vi "Exp11.vi"() -> ()   [LabVIEW 2009]
uses:
  <vilib>/Simulation/Scripting/Companion Diagram/SimConfigNode/SimDog.xnode
  <vilib>/Simulation/Scripting/Companion Diagram/SimConfigNode/SimParams.ctl
  <vilib>/Simulation/Scripting/Companion Diagram/SimConfigNode/_simSolvers.ctl
  <vilib>/Simulation/Implementation/Shared/SIMSCR Execution Mode.ctl
  <vilib>/Simulation/Implementation/Shared/SIM Bundle Sim Info.vi
  <vilib>/Simulation/Implementation/Shared/NILVSim_GetModelError.vi
  <vilib>/Simulation/Implementation/Shared/SIM Unbundle Sim Info.vi
  <vilib>/Platform/TimedLoop/XDataNode/XDataNode.xnode
  <vilib>/Platform/TimedLoop/XDataNode/loadlvalarms.vi
  <vilib>/Platform/TimedLoop/XDataNode/timing_clust.ctl
  <vilib>/Platform/TimedLoop/XDataNode/nitl_modes.ctl
  <vilib>/Platform/TimedLoop/XDataNode/wakeup.ctl
  <vilib>/Simulation/Implementation/Shared/NILVSim_Initialize.vi
  <vilib>/Simulation/Implementation/Shared/NILVSim_FinishedLate.vi
  <vilib>/Simulation/Implementation/Shared/NILVSim_Manager.vi
  <vilib>/Simulation/Scripting/Editor Utilities/SIM subVI tag data.ctl
  <vilib>/Simulation/Scripting/Editor Utilities/SIM subVI execution type.ctl
  <vilib>/Simulation/Utility/SIMX Halt/SIMX Halt.xnode
  <vilib>/Simulation/Utility/Implementation/SIM Halt.vi
  <vilib>/Simulation/Implementation/Shared/SIM Fire Discrete SubVI.vi
  <vilib>/Simulation/SignalArithmetic/SIMX Gain/SIMX Gain.xnode
  <vilib>/Simulation/SignalArithmetic/Implementation/NILVSim Gain.llb/SIM Gain (scalar).vi
  <vilib>/Simulation/SignalArithmetic/SIMX Summation/SIMX Summation.xnode
  <vilib>/Simulation/Nonlinear/SIMX Saturation/SIMX Saturation.xnode
  <vilib>/Simulation/Nonlinear/Implementation/NILVSim Saturation.llb/SIM Saturation (scalar).vi
  <vilib>/Simulation/Implementation/Shared/NILVSim_FinalizeModel.vi
  Instance           8 13Saved   Exp10 .vi
  Instance           9 13Saved   Exp10 .vi
  Instance          10 13Saved   Exp10 .vi
  Instance          11 13Saved   Exp10 .vi
  <vilib>/Platform/TimedLoop/XDataNode/XDNodeRunTimeDep.lvlib
panel:
  in  "Controlador":cluster{"Kc":dbl, "Kaux":dbl}
  in  "stop":bool
  in  "Set-Point":T1={"Magnitude"=5.0, "Frequência"=0.02, "Offset"=2.5}
  in  "Set-point:\nMan / Auto":bool
  out "Medidas":dbl[][](graph)
  in  "AO0\n(manual)":dbl(slide) scale=-10.0..10.0
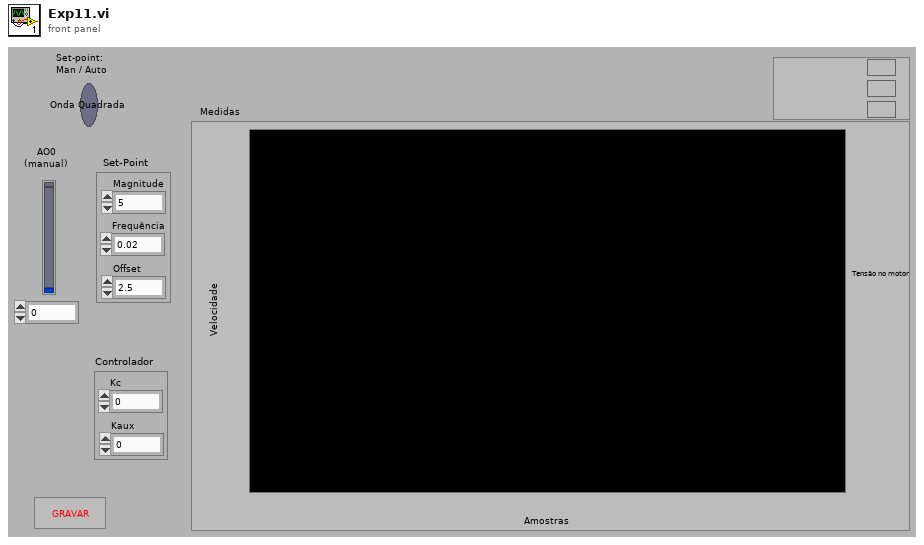
[diagram p1: front panel]
types:
  T1 = cluster{"Magnitude":dbl, "Frequência":dbl, "Offset":dbl}
  T2 = typedef "SIM subVI tag data.ctl" = cluster{"period":dbl, "skew":dbl, "Simulation execution type":T3}
  T3 = typedef "SIM subVI execution type.ctl" = enum16{"Function call", "Discrete", "Continuous", "Initialization only", "Final step only"}
  T4 = typedef "XDNodeRunTimeDep.lvlib/timing_clust.ctl" = cluster{"Expected End [f-1]":u64, "Actual End [f-1]":u64, "Finished Late? [f-1]":bool, "Expected End [i-1]":u64, "Actual End [i-1]":u64, "Finished Late? [i-1]":bool, "Expected Start [i]":u64, "Actual Start [i]":u64, "Expected Start [f]":u64, "Actual Start [f]":u64, "Source Name":string, "Structure Name":string, "Period":i64, "Deadline":i64, "Offset":i64, "Start":i64, "Priority":i32, "Timeout":i32, "Mode":T5, "Wakeup Reason":T6, "Error":errorcluster, "Source Type":string, "Secondary Source Type":string, "Global End Time":u64, "Global Start Time":u64, "Frame Duration":u64, "Iteration Duration":u64, "Assigned CPU":i32, "I/O Scan Engine Mode":u32}
  T5 = typedef "XDNodeRunTimeDep.lvlib/nitl_modes.ctl" = enum32{"No Change", "Process missed periods, maintain original phase", "Discard missed periods, maintain original phase", "Process missed periods, ignore original phase", "Discard missed periods, ignore original phase"}
  T6 = typedef "XDNodeRunTimeDep.lvlib/wakeup.ctl" = enum32{"Normal", "Aborted", "Asynchronous wakeup", "Timing source error", "Timed loop error", "Timeout"}
  T7 = typedef "SimParams.ctl" = cluster{"Initial Time (s)":dbl, "Final Time (s)":dbl, "Step Size (s)":dbl, "ODE Solver":T8, "Minimum Step Size (s)":dbl, "Maximum Step Size (s)":dbl, "Relative Tolerance":dbl, "Absolute Tolerance":dbl, "Software Timing":bool, "Initial Step Size (s)":dbl, "Automatic Fixed Step Size?":bool, "Automatic Discrete Step Size?":bool, "Discrete Step Size (s)":dbl, "Calculate using Time Step":bool, "Solver Wired?":bool, "Prev.Frm.Expected End":u64, "Prev.Frm.Actual End":u64, "Prev.Frm.Finished Late?":bool, "Prev.Iter.Expected End":u64, "Prev.Iter.Actual End":u64, "Prev.Iter.Finished Late?":bool, "Expected Iteration Start":u64, "Actual Iteration Start":u64, "Expected Frame Start":u64, "Actual Frame Start":u64, "Source Name":string, "Name":string, "Period":i64, "Deadline":i64, "Offset":i64, "Start":i64, "Priority":i32, "Timeout":i32, "Processor":i32, "Mode":enum32{"No Change", "Process missed periods, maintain original phase", "Discard missed periods, maintain original phase", "Process missed periods, ignore original phase", "Discard missed periods, ignore original phase"}, "Wakeup reason":enum32{"Normal", "Aborted", "Asynchronous wakeup", "Timing source error", "Timed loop error", "Timeout"}, "Error":errorcluster, "Source Type":string, "Secondary Source Type":string, "Global End Time":u64, "Global Start Time":u64, "Full Solver Reset":bool, "Execution Mode":T9, "Nan/Inf Check":bool, "Custom Solver Library":string, "Solver Is Variable":bool, "custom solver name":string}
  T8 = typedef "_simSolvers.ctl" = enum16{"Runge-Kutta 1 (Euler)", "Runge-Kutta 2", "Runge-Kutta 3", "Runge-Kutta 4", "Runge-Kutta 23 (variable)", "Runge-Kutta 45 (variable)", "BDF (variable)", "Adams-Moulton (variable)", "Rosenbrock (variable)", "Discrete States Only", "Linearizer", "State Query", "Trim Eval", "Custom Solver"}
  T9 = typedef "SIMSCR Execution Mode.ctl" = u16
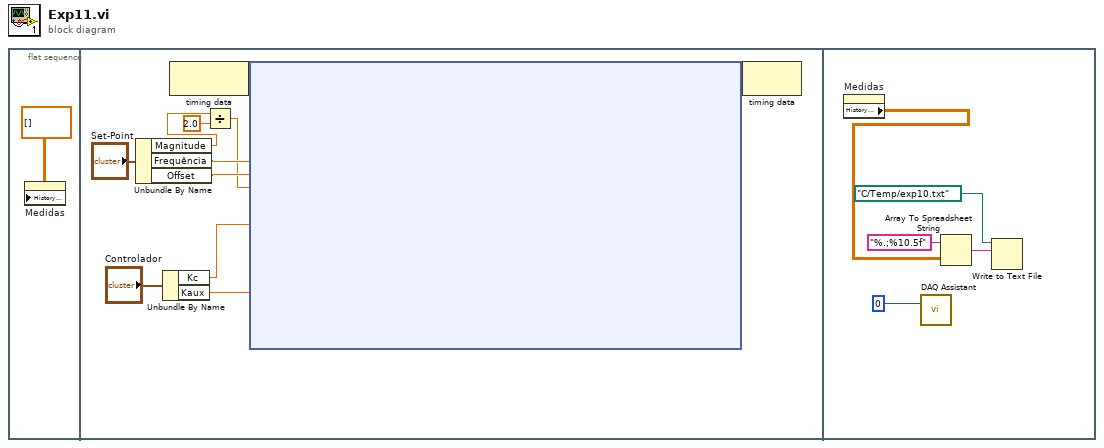
[diagram p0: block diagram]
diagram:
  n1 = flat-sequence {
    frame #0 {
      n2 = property on="Medidas" class="WFChart (strict)"("History Data"=dbl[][] []) -> ()  [unwired: 2 in, 2 out]
    }
    frame #1 {
      n3 = Unbundle By Name("Set-Point") -> ("Magnitude"=w7:dbl, "Frequência"=w9:dbl, "Offset"=w8:dbl)
      n4 = Unbundle By Name("Controlador") -> ("Kc"=w3:dbl, "Kaux"=w2:dbl)
      n5 = node-c288() -> (w12:variant)  [unwired: 1 in]
      n6 = Divide(x=w7, y=2.0) -> (x/y=w5:dbl)
      n7 = node-c254 ("Control & Simulation Loop")(w12, w9, w8, w5, w3, w2) -> (w11:variant)
      n8 = node-c288(w11) -> ()  [unwired: 1 out]
    }
    frame #2 {
      n9 = property on="Medidas" class="WFChart (strict)"() -> ("History Data"=w277:dbl[][])  [unwired: 2 in, 2 out]
      n10 = call "DAQ Assistant"("data"=0) -> ()  [unwired: 17 in, 2 out]
      n11 = Array To Spreadsheet String(array=w277, 3:"%.;%10.5f" ("format string")) -> (spreadsheet string=w280:string)  [unwired: 1 in]
      n12 = Write to Text File(file (use dialog)=path "C:/Temp/exp10.txt", text=w280) -> ()  [unwired: 2 in, 3 out]
    }
  }
